vi "CRYReplace Message Curve Name.vi"(8 "Type In":string, 11 "Setup in":T1={"No.VI"=0, "Category"="", "StepName"="", "Seq setup flattened"="", "Comment"="", "Steps config."=[], "Jump config"=[], "Start"=0.0, "Increment"=0.0, "Name"="Pa", "Unit"="Pa", "Y data"=1, "Y prefix"="", "Y dB ref"=1.0, "Y unit"="", "Repeat State Array"=[]} {"Repeat State Array"."Start" format="%#_5g"; "Y dB ref" format="%.1f"; "Y data" items=["dB", "Lin"]; "Start" format="%#_5g"}) -> ()   [LabVIEW 2013]
uses:
  Typedef Control/CRYData Cluster.ctl
  Typedef Control/CRYWaveform Cluster.ctl
  Typedef Control/CRYStep.ctl
panel:
  out "Inserted Names Out":string[](array[string])
  out "Types Out":string[](array[string])
  in  "Step name":string
  out "Wave out":T2[](array[typedef]) {"Y dB ref" format="%.1f"; "Y axis" items=["Log", "Lin"]; "Y data" items=["dB", "Lin"]; "X data" items=["dB", "Lin"]}
  out "Data Out":T3[](array[typedef]) {"Z data" items=["dB", "Lin"]; "X data" items=["dB", "Lin"]; "Y data" items=["dB", "Lin"]; "Z dB ref" format="%.1f"; "Z axis" items=["Log", "Lin"]; "X dB ref" format="%.1f"; "X axis" items=["Log", "Lin"]; "Y axis" items=["Log", "Lin"]; "Y dB ref" format="%.1f"; "Curve"."z" format="%.2f"; "Curve"."y" format="%.2f"; "Curve"."x" format="%.2f"}
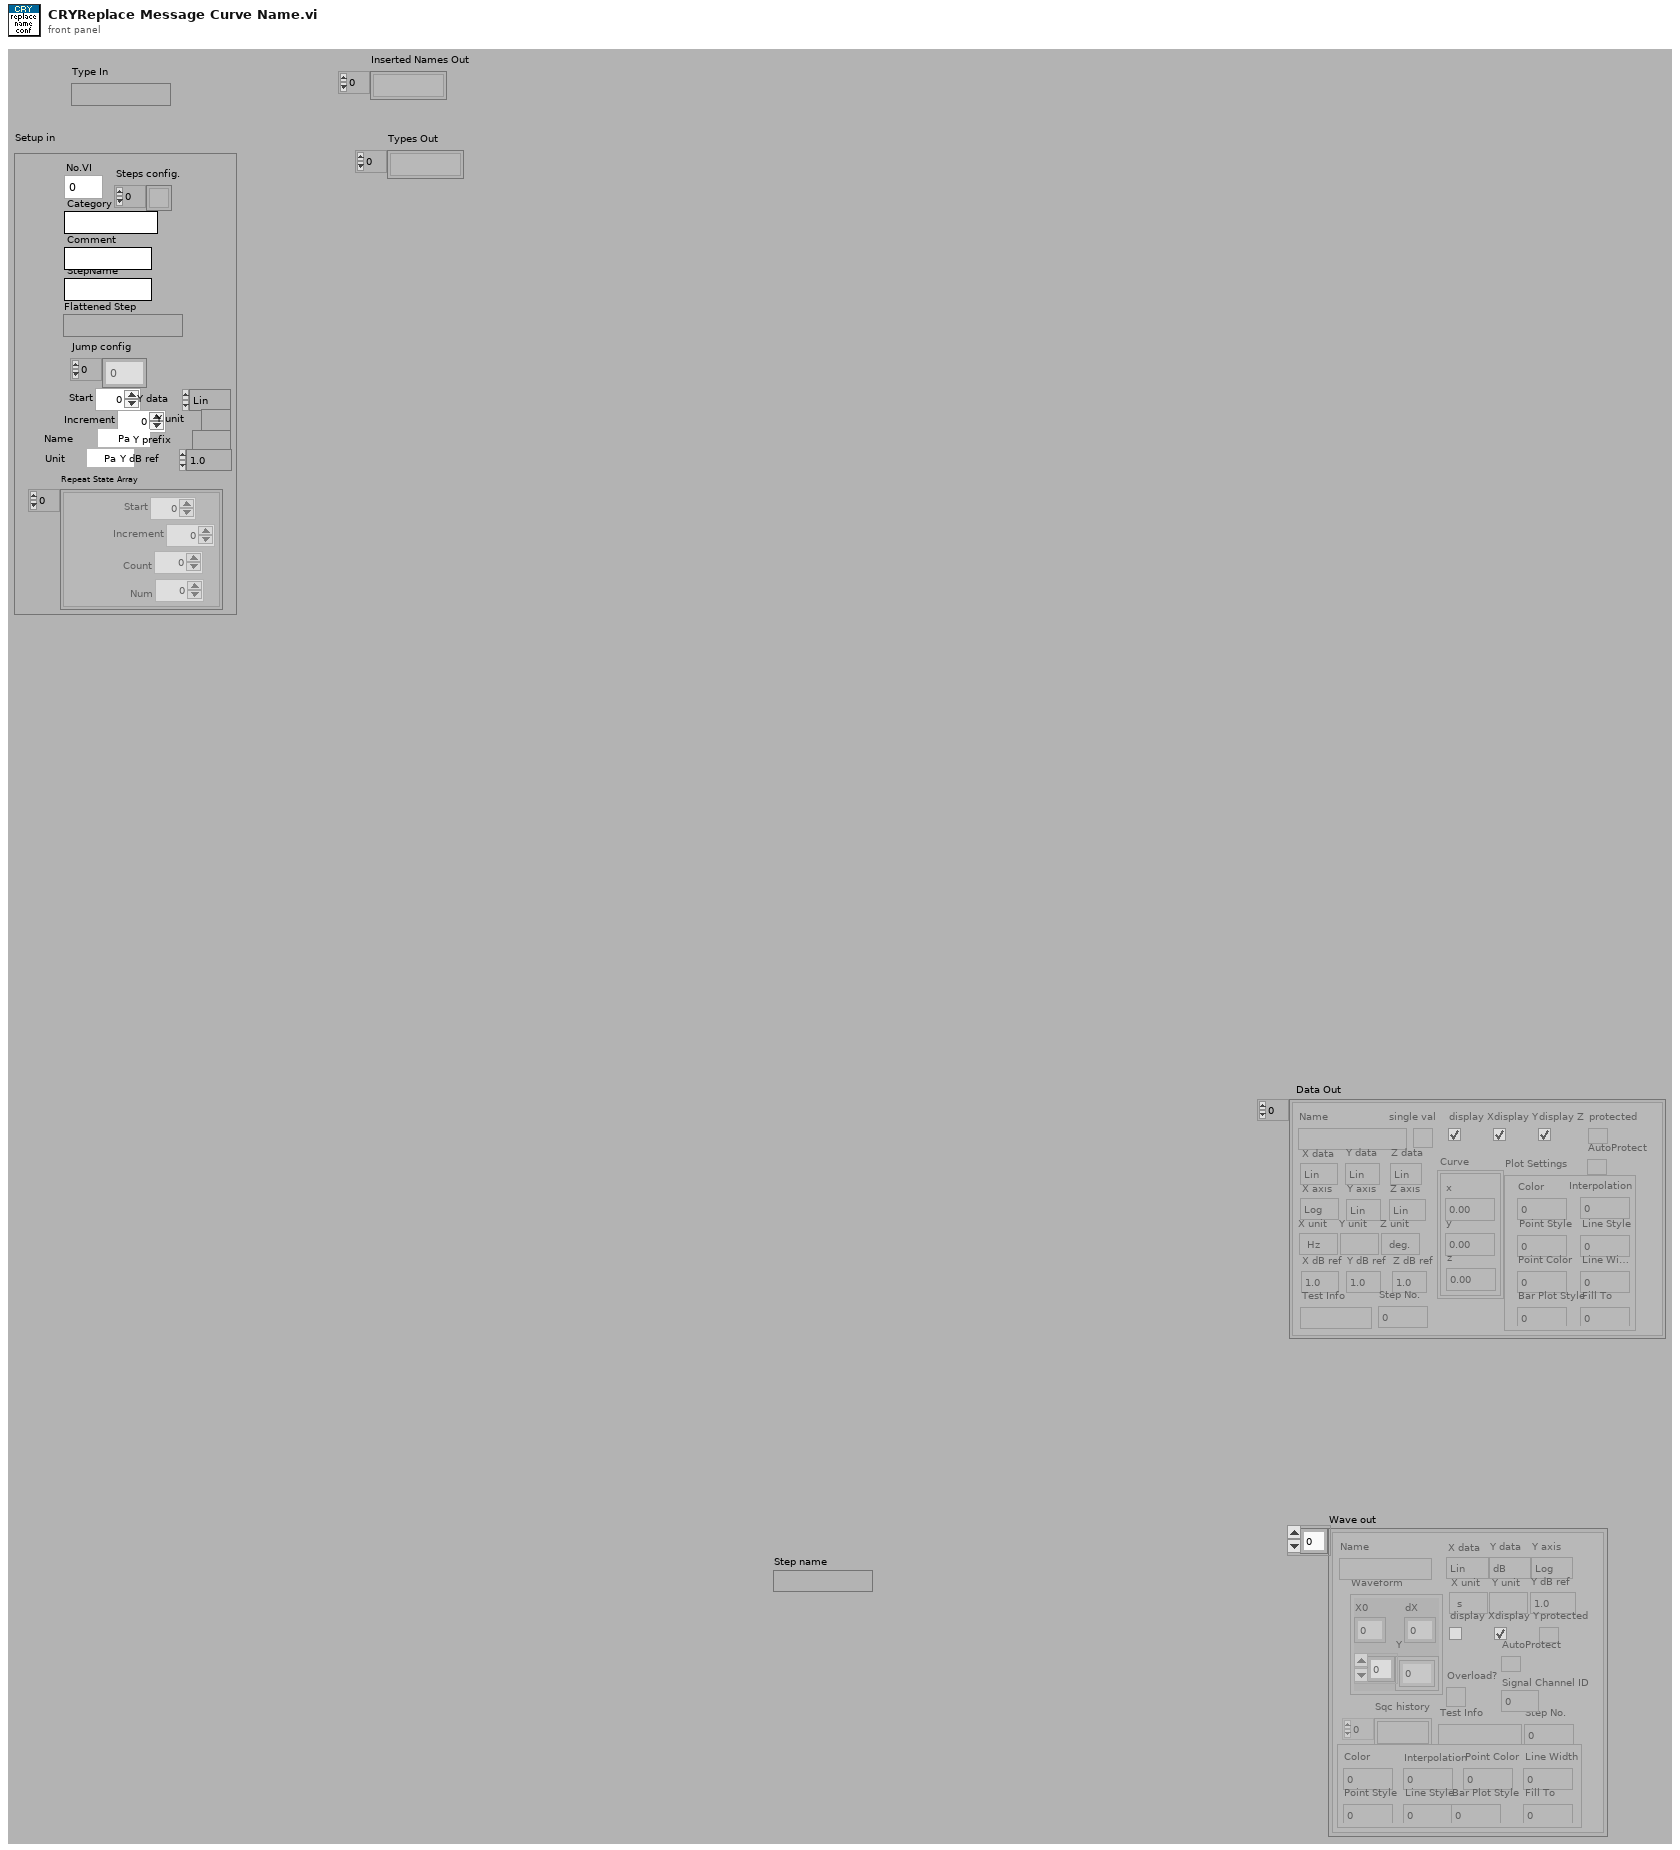
[diagram p1: front panel]
types:
  T1 = typedef "CRYStep.ctl" = cluster{"No.VI":i32, "Category":string, "StepName":string, "Seq setup flattened":string, "Comment":string, "Steps config.":bool[], "Jump config":i32[], "Start":dbl, "Increment":dbl, "Name":string, "Unit":string, "Y data":u16, "Y prefix":string, "Y dB ref":dbl, "Y unit":string, "Repeat State Array":cluster{"Start":dbl, "Increment":dbl, "Count":i32, "Num":i32}[]}
  T2 = typedef "CRYWaveform Cluster.ctl" = cluster{"Waveform":cluster{"X0":dbl, "dX":dbl, "Y":sgl[]}, "X data":u16, "Y data":u16, "Y axis":u16, "X unit":string, "Y unit":string, "Y dB ref":dbl, "display Y":bool, "display X":bool, "Overload?":bool, "Test Info":string, "Step No.":i32, "Name":string, "protected":bool, "Sqc history":string[], "Signal Channel ID":i32, "Plot Settings":cluster{"Color":u32, "Interpolation":u8, "Point Style":u8, "Line Style":u8, "Point Color":u32, "Line Width":u8, "Bar Plot Style":u8, "Fill To":i16}, "AutoProtect":bool}
  T3 = typedef "CRYData Cluster.ctl" = cluster{"Name":string, "Curve":cluster{"x":dbl, "y":dbl, "z":dbl}[], "X data":u16, "Y data":u16, "Z data":u16, "X axis":u16, "Y axis":u16, "Z axis":u16, "X unit":string, "Y unit":string, "Z unit":string, "X dB ref":dbl, "Y dB ref":dbl, "Z dB ref":dbl, "single val":bool, "protected":bool, "display X":bool, "display Y":bool, "display Z":bool, "Test Info":string, "Step No.":i32, "Plot Settings":cluster{"Color":u32, "Interpolation":u8, "Point Style":u8, "Line Style":u8, "Point Color":u32, "Line Width":u8, "Bar Plot Style":u8, "Fill To":i16}, "AutoProtect":bool}
  T4 = cluster{"Start":dbl, "Increment":dbl, "Count":i32, "Num":i32}[]
  T5 = typedef "CRYMessages Cluster.ctl" = cluster{"Name":string, "Type":u16, "Command Msg":string, "Flags":u16, "Dialog?":bool, "Numeric?":bool, "Wait?":bool, "Pause [ms]":i32, "pattern":u32, "Address":string, "Operation":i32, "bytes":i32, "Line selected":u32, "RS232 Func":u16, "Serial Ctrl lines":u16, "Interf #":u8, "GPIB func":u16, "GPIB cmd":u16, "GPIB rem en":bool, "GPIB term":i32, "Curves generated":string[], "Units":cluster{"unit":string, "dB ref":dbl, "axis":u16, "data":u16, "Common dB ref.":u16}, "Axis":u16, "Default Value":dbl, "Message Tilte":string, "Port #":i32, "Print Unit":string, "Text Format":cluster{"Size":u32, "Plain":bool, "Bold":bool, "Italic":bool, "Underline":bool, "Strikethrough":bool, "Color":u32, "Font":string}, "Help":string, "Tab Value":enum32{"Setting", "Help"}, "pattern 2":u32, "Line selected 2":u32, "H_Bits":cluster{"Bits":string[], "Invert":bool, "All":bool}[], "G_Bits":cluster{"Bits":string[], "Invert":bool, "All":bool}[]}
  T6 = typedef "CRYResult Cluster.ctl" = cluster{"Name":string, "Margin":dbl, "unit":string, "Verdict":bool, "Limit":string, "Max/Min":string, "protected":bool, "Step No.":i32, "Test Info":string, "AutoProtect":bool}
  T7 = cluster{"unit":string, "dB ref":dbl, "axis":u16, "data":u16, "Common dB ref.":u16}
  T8 = cluster{"Numeric Entry":dbl, "Numeric Entry":dbl, "Numeric Entry":dbl}
  T9 = cluster{"Numeric":dbl, "Numeric":dbl, "Numeric":dbl}
  T10 = cluster{"Numeric Entry":dbl, "Numeric Entry":dbl, "Numeric Entry":dbl}[]
  T11 = typedef "CRYData Cluster Array.ctl" = T3[]
  T12 = typedef "CRYResult Cluster Array.ctl" = T6[]
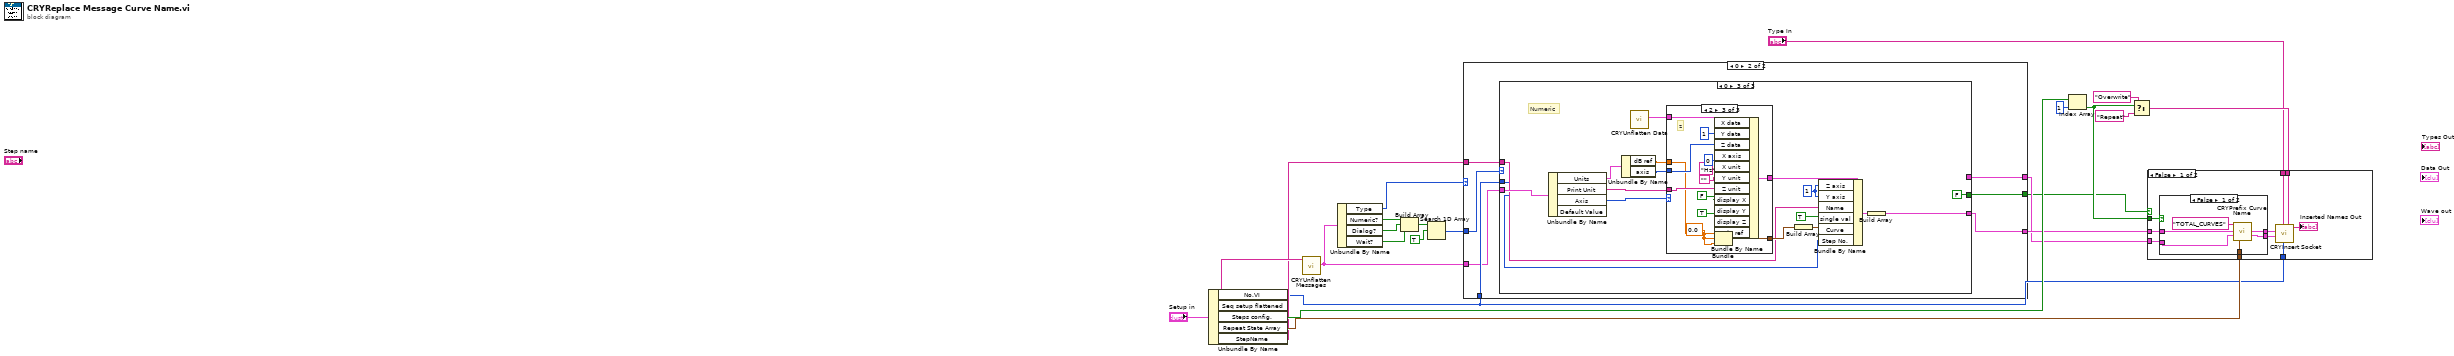
[diagram p0: block diagram]
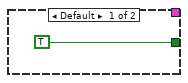
[diagram p2: hidden frame]
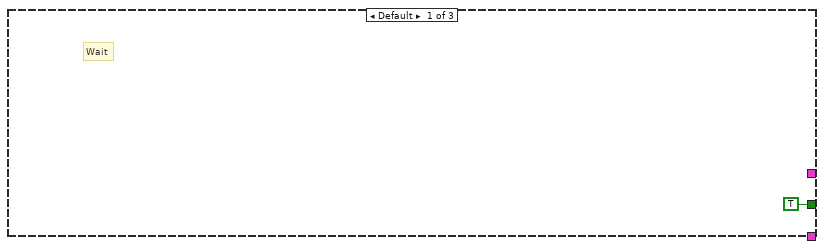
[diagram p3: hidden frame]
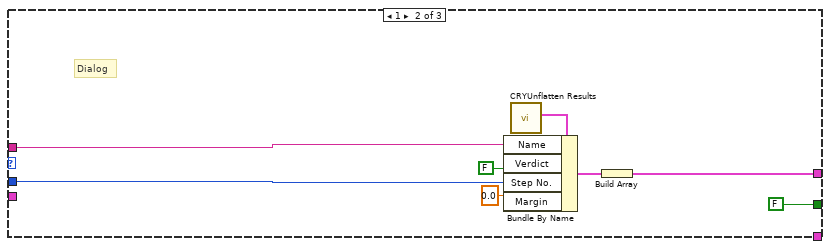
[diagram p4: hidden frame]
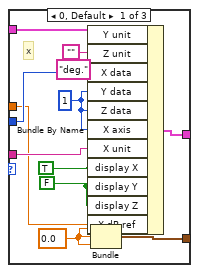
[diagram p5: hidden frame]
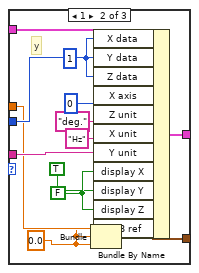
[diagram p6: hidden frame]
diagram:
  n1 = Unbundle By Name("Setup in") -> ("No.VI"=w12:i32, "Seq setup flattened"=w22:string, "Steps config."=w15:bool[], "Repeat State Array"=w16:T4, "StepName"=w13:string)
  n2 = call "CRYUnflatten Messages.vi"("Unflatten Messages"=w22) -> ("Messages"=w11:T5)  [unwired: 10 out]
  n3 = Unbundle By Name(w11) -> ("Type"=w2:u16, "Numeric?"=w8:bool, "Dialog?"=w7:bool, "Wait?"=w6:bool)
  n4 = Build Array(w8, w7, w6) -> (w5:bool[])
  n5 = Search 1D Array(1D array=w5, element=TRUE) -> (index of element=w3:i32)  [unwired: 1 in]
  n6 = case shown="0" w2 {
    tunnel: w13 -> [_ w31]
    tunnel: w12 -> [_ w30]
    tunnel: w11 -> [_ w29]
    tunnel: [_ w28] -> w10
    tunnel: [_ w27] -> w9
    tunnel: w3 -> [_ w26]
    tunnel: [TRUE ("element") w25] -> w1
    frame Default {
    }
    frame 0 {
      n7 = case shown="0" w26 {
        tunnel: [_ w36 _] -> w27
        tunnel: w31 -> [_ w35 w44]
        tunnel: w30 -> [_ w34 w43]
        tunnel: w29 -> [_ _ w45]
        tunnel: [_ _ w42] -> w28
        tunnel: [TRUE ("element") FALSE ("element") FALSE ("element")] -> w25
        frame Default {
          # "Wait"
        }
        frame 1 {
          # "Dialog"
          n8 = call "CRYUnflatten Results.vi"() -> ("Result"=w40:T6)  [unwired: 9 in, 2 out]
          n9 = Bundle By Name(cluster=w40, "Name"=w35, "Verdict"=FALSE ("NewVal"), "Step No."=w34, "Margin"=0.0) -> (w39:T6)
          n10 = Build Array(w39) -> (w36:T6[])
        }
        frame 0 {
          w51 = u16 1 ("Z axis")
          # "Numeric"
          n11 = Unbundle By Name(w45) -> ("Units"=w53:T7, "Print Unit"=w54:string, "Axis"=w55:u16)  [unwired: 1 out]
          n12 = Unbundle By Name(w53) -> ("dB ref"=w56:dbl, "axis"=w52:u16)
          n13 = call "CRYUnflatten Data.vi"() -> ("Datum"=w47:T3)  [unwired: 1 in, 10 out]
          n14 = case shown="2" w55 {
            tunnel: [w69 w82 w95] -> w48
            tunnel: w47 -> [w68 w81 w94]
            tunnel: [w67 w80 w93] -> w46
            tunnel: w54 -> [w66 w79 w92]
            tunnel: w52 -> [w60 w74 w86]
            tunnel: w56 -> [w59 w71 w84]
            frame 0, Default {
              w63 = u16 1 ("Y data")
              w64 = FALSE ("display Y")
              w58 = 0.0 ("Numeric Entry")
              # "x"
              n15 = Bundle By Name(cluster=w68, "Y unit"="", "Z unit"="deg.", "X data"=w60, "Y data"=w63, "Z data"=w63, "X axis"=w63, "X unit"=w66, "display X"=TRUE, "display Y"=w64, "display Z"=w64, "X dB ref"=w59) -> (w67:T3)
              n16 = Bundle("Numeric Entry"=w58, "Numeric Entry"=w58, "Numeric Entry"=w58) -> (w69:T8)  [unwired: 1 out]
            }
            frame 1 {
              w70 = 0.0 ("Numeric")
              w73 = u16 1 ("X data")
              w78 = FALSE ("display X")
              # "y"
              n17 = Bundle("Numeric"=w70, "Numeric"=w70, "Numeric"=w70) -> (w82:T9)  [unwired: 1 out]
              n18 = Bundle By Name(cluster=w81, "X data"=w73, "Y data"=w74, "Z data"=w73, "X axis"=u16 0, "Z unit"="deg.", "X unit"="Hz", "Y unit"=w79, "display X"=w78, "display Y"=TRUE, "display Z"=w78, "Y dB ref"=w71) -> (w80:T3)
            }
            frame 2 {
              w85 = u16 1 ("X data")
              w91 = FALSE ("display X")
              w83 = 0.0 ("Numeric Entry")
              # "z"
              n19 = Bundle By Name(cluster=w94, "X data"=w85, "Y data"=w85, "Z data"=w86, "X axis"=u16 0, "X unit"="Hz", "Y unit"="", "Z unit"=w92, "display X"=w91, "display Y"=w91, "display Z"=TRUE, "Z dB ref"=w84) -> (w93:T3)
              n20 = Bundle("Numeric Entry"=w83, "Numeric Entry"=w83, "Numeric Entry"=w83) -> (w95:T8)  [unwired: 1 out]
            }
          }
          n21 = Build Array(w48) -> (w50:T10)
          n22 = Bundle By Name(cluster=w46, "Z axis"=w51, "Y axis"=w51, "Name"=w44, "single val"=TRUE ("Bundle Element"), "Curve"=w50, "Step No."=w43) -> (w57:T3)
          n23 = Build Array(w57) -> (w42:T3[])
        }
      }
    }
  }
  n24 = Index Array(array=w15, index=1) -> (element=w17:bool)
  n25 = Select(t="Overwrite" ("Y unit"), s=w17, f="Repeat") -> (s? t:f=w18:string)
  n26 = case shown="False" w1 {
    tunnel: w18 -> [w103 _]
    tunnel: w16 -> [w102 _]
    tunnel: "Type In" -> [w101 _]
    tunnel: w10 -> [w99 _]
    tunnel: w9 -> [w98 _]
    tunnel: w17 -> [w97 _]
    tunnel: w12 -> [w96 _]
    frame False {
      n27 = case shown="False" w97 {
        tunnel: w99 -> [w111 w113]
        tunnel: w98 -> [w110 w112]
        tunnel: [w109 w112] -> w105
        tunnel: [w108 w113] -> w104
        tunnel: w102 -> [w107 _]
        frame False {
          n28 = call "CRYPrefix Curve Name.vi"("Type In"="TOTAL_CURVES", "Values In"=w111, "Results In"=w110, "Repeat State Array In"=w107) -> ("Values Out"=w108:T11, "Results Out"=w109:T12)  [unwired: 8 in, 2 out]
        }
        frame True {
        }
      }
      n29 = call "CRYInsert Socket.vi"("sOption2"=w103, "Step No."=w96, "sOption1"=w101, "Results"=w105, "Values"=w104) -> ("Inserted Names Out"=→"Inserted Names Out":string[])  [unwired: 6 in]
    }
    frame True {
    }
  }
